vi "Plugin.Shutdown.vi"(8 "error in (no error)":errorcluster, 11 "UDP Plugin in":refnum<class "UDP Plugin.lvclass">) -> (0 "error out":errorcluster, 3 "UDP Plugin out":refnum<class "UDP Plugin.lvclass">)   [LabVIEW 2017, in "UDP Plugin.lvclass"]
uses:
  UDP Plugin.lvclass
  Plugin.lvclass
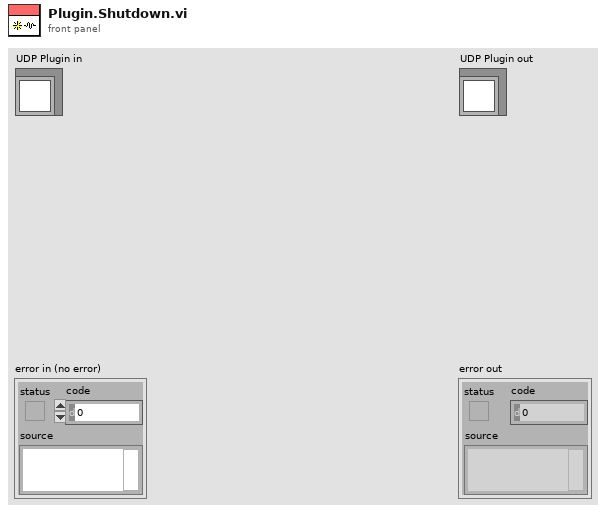
[diagram p1: front panel]
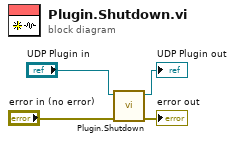
[diagram p0: block diagram]
diagram:
  n1 = call-parent "Plugin.Shutdown.vi"("error in (no error)"="error in (no error)", "Plugin in"="UDP Plugin in") -> ("error out"=→"error out":errorcluster, "Plugin out"=→"UDP Plugin out":refnum<class "UDP Plugin.lvclass">)  [unwired: 8 in]
